vi "to string array.vi"(8 "error in (no error)":errorcluster, 11 "module configuration in":refnum<class "Scan Engine configuration.lvclass">) -> (0 "error out":errorcluster, 1 "Array":string[][](array[string]), 2 "version":string, 3 "module configuration out":refnum<class "Scan Engine configuration.lvclass">)   [LabVIEW 2015, in "Scan Engine configuration.lvclass"]
uses:
  Scan Engine configuration.lvclass
  Scan Engine configuration.lvclass/Scan Engine configuration.ctl
  <vilib>/NI/Tag Bus/tag/tag descriptor.lvclass/tag descriptor.ctl
  <vilib>/NI/Tag Bus Module Framework/channel/TBM channel.lvclass/TBM channel.ctl
  Read Lines.vi
  <vilib>/NI/Tag Bus Module Framework/channel/TBM channel.lvclass
  editor node/Scan Engine editor node.lvclass
  <vilib>/NI/Tag Bus/tag/tag descriptor.lvclass
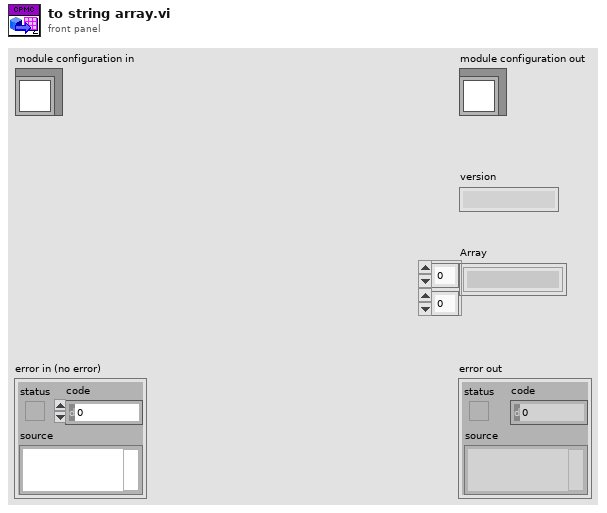
[diagram p1: front panel]
types:
  T1 = typedef "Scan Engine configuration.lvclass/Line.ctl" = cluster{"channel":refnum<class "TBM channel.lvclass">, "Tag":string}
  T2 = typedef "TBM channel.lvclass/channel classification.ctl" = enum16{"input data", "output data", "processing parameter", "processing result"}
  T3 = typedef "tag bus.lvlib/tag descriptor.lvclass/Data Type.ctl" = enum16{"Double", "Single", "I64", "I32", "I16", "I8", "U64", "U32", "U16", "U8", "Boolean", "String", "Array of Double", "Array of Single", "Array of I64", "Array of I32", "Array of I16", "Array of I8", "Array of U64", "Array of U32", "Array of U16", "Array of U8", "Array of Boolean", "Array of String"}
  T4 = typedef "Scan Engine editor node.lvclass/permissions.ctl" = enum32{"Read from HW", "Write to HW"}
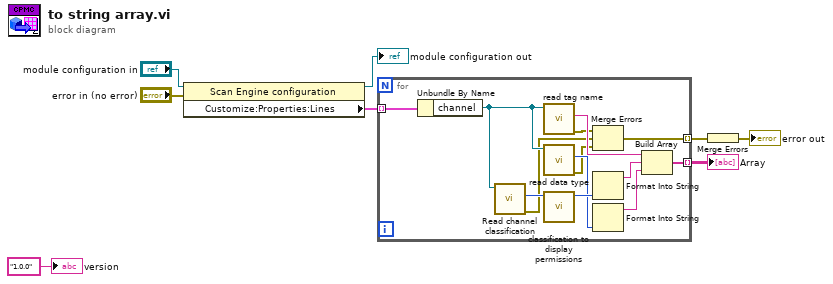
[diagram p0: block diagram]
diagram:
  n1 = property class="Scan Engine configuration"(reference="module configuration in", error in="error in (no error)") -> (reference out=→"module configuration out":refnum<class "Scan Engine configuration.lvclass">, "Customize:Properties:Lines"=w6:T1[])  [unwired: 1 out]
  n2 = for {
    tunnel: w6 -> [w21] mode=indexing
    tunnel: [w13] -> w5 mode=indexing
    tunnel: [w9] -> w2 mode=indexing
    n3 = Unbundle By Name(w21) -> ("channel"=w16:refnum<class "TBM channel.lvclass">)
    n4 = call <vilib>:"Read channel classification.vi"("channel in"=w16) -> ("error out"=w11:errorcluster, "channel classification"=w19:T2)  [unwired: 8 in, 1 out]
    n5 = call <vilib>:"read tag name.vi"("system tag in"=w16) -> ("error out"=w12:errorcluster, "name"=w20:string)  [unwired: 8 in, 1 out]
    n6 = call <vilib>:"read data type.vi"("system tag in"=w16) -> ("error out"=w10:errorcluster, "data type"=w15:T3)  [unwired: 8 in, 1 out]
    n7 = call "classification to display permissions.vi"("channel classification"=w19) -> ("permissions"=w18:T4)  [unwired: 10 in]
    n8 = Merge Errors(w12, w11, w10) -> (w9:errorcluster)
    n9 = Format Into String(w18) -> (resulting string=w17:string)  [unwired: 3 in, 1 out]
    n10 = Format Into String(w15) -> (resulting string=w14:string)  [unwired: 3 in, 1 out]
    n11 = Build Array(w20, w17, w14) -> (w13:string[])
  }
  "Array" <- w5
  n12 = Merge Errors(w2) -> (→"error out":errorcluster)
  "version" <- "1.0.0" ("version")
